vi "Read States.vi"(8 "error in (no error)":errorcluster, 11 "PenaltyAttackTacticVSS in":refnum<class "PenaltyAttackTacticVSS.lvclass">) -> (0 "error out":errorcluster, 2 "States":enum16{"PenaltyPos", "Exit"}(ring), 3 "PenaltyAttackTacticVSS out":refnum<class "PenaltyAttackTacticVSS.lvclass">)   [LabVIEW 2018, in "PenaltyAttackTacticVSS.lvclass"]
uses:
  PenaltyAttackTacticVSS.lvclass
  PenaltyAttackTacticVSS.lvclass/PenaltyAttackTacticVSS.ctl
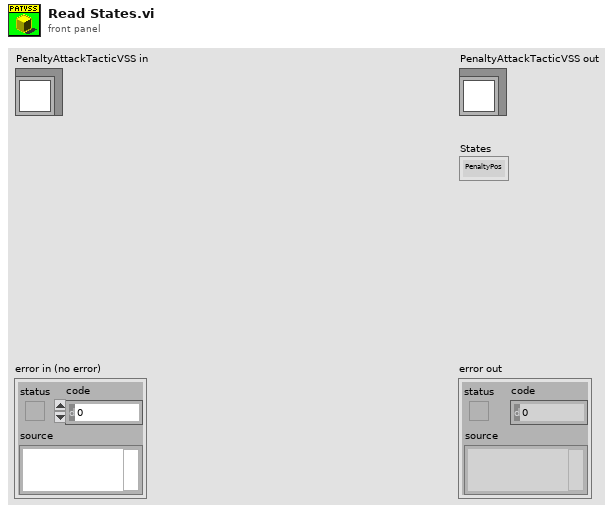
[diagram p1: front panel]
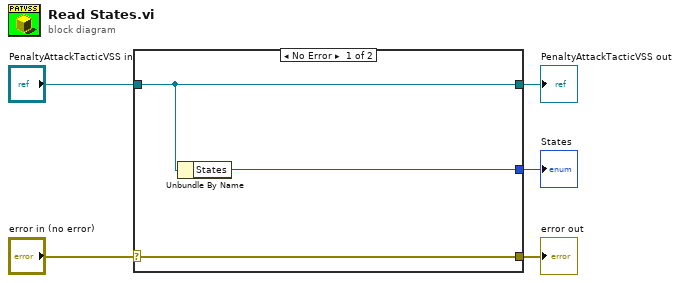
[diagram p0: block diagram]
diagram:
  n1 = case shown="No Error" "error in (no error)" {
    selector: "error in (no error)" -> [w8 w9]
    tunnel: [w8 w9] -> w4
    tunnel: [w7 w10] -> w2
    tunnel: "PenaltyAttackTacticVSS in" -> [w7 w10]
    tunnel: [w6 _] -> w1
    frame No Error {
      n2 = Unbundle By Name(w7) -> ("States"=w6:enum16{"PenaltyPos", "Exit"})
    }
    frame Error {
    }
  }
  "error out" <- w4
  "PenaltyAttackTacticVSS out" <- w2
  "States" <- w1
